vi "ConvertTdmsFileToNoDaqMxRaw.vi"() -> ()   [LabVIEW 2014]
panel:
  in  "转换总数":i64
  in  "偏移量":i64
  out "error":errorcluster
  in  "Convert":bool
  in  "Stop Button":bool
  in  "File With RawDaq":path
  in  "New File":path
  # "Very simple utility to read in a TDMS file and the write out to a new TDMS file.\nThis will strip out DAQmxRaw data which is problematic for reading with other tools."
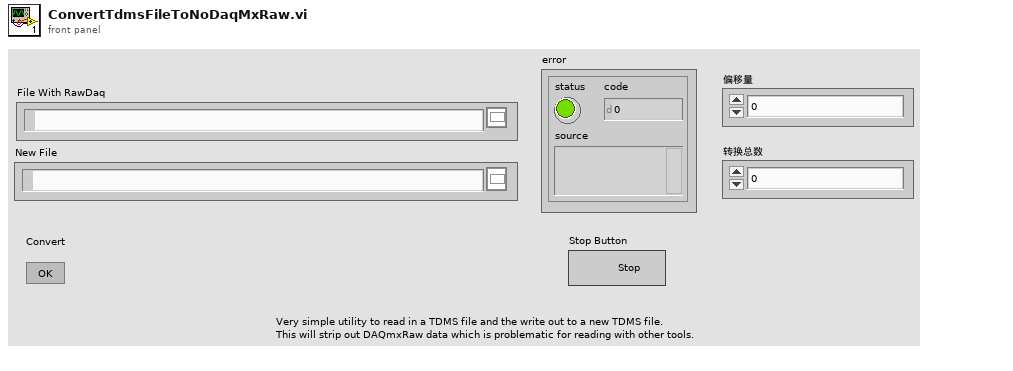
[diagram p1: front panel]
types:
  T1 = enum16{"open", "open or create", "create or replace", "create", "open (read-only)"}
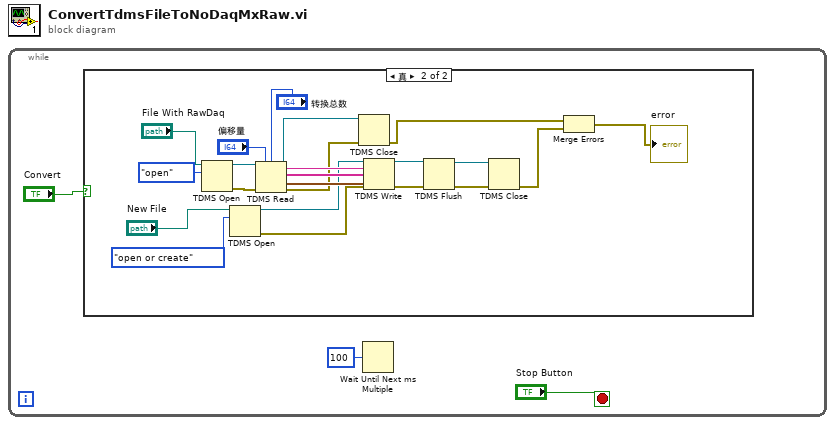
[diagram p0: block diagram]
diagram:
  n1 = while {
    stop <- "Stop Button" stop-if-true
    n2 = case shown="真" "Convert" {
      frame False {
      }
      frame True {
        n3 = TDMS Open(10:T1."open" ("operation (0:open)"), 11:"File With RawDaq") -> (0:w21:errorcluster, 3:w22:refnum<k34>)  [unwired: 5 in]
        n4 = TDMS Open(10:T1."open or create" ("operation (0:open)"), 11:"New File") -> (0:w9:errorcluster, 3:w18:refnum<k34>)  [unwired: 5 in]
        n5 = TDMS Read(0:w22, 1:"偏移量", 2:"转换总数", 11:w21) -> (4:w14:refnum<k34>, 6:w25:string, 8:w24:string[], 10:w23:waveform(dbl)[], 15:w15:errorcluster)  [unwired: 4 in, 1 out]
        n6 = TDMS Close(8:w15, 11:w14) -> (0:w8:errorcluster)  [unwired: 1 out]
        n7 = TDMS Write(0:w18, 5:w25, 7:w24, 9:w23, 11:w9) -> (4:w12:refnum<k34>, 15:w13:errorcluster)  [unwired: 1 in, 2 out]
        n8 = TDMS Flush(4:w13, 7:w12) -> (0:w11:errorcluster, 3:w10:refnum<k34>)
        n9 = TDMS Close(8:w11, 11:w10) -> (0:w7:errorcluster)  [unwired: 1 out]
        n10 = Merge Errors(w8, w7) -> (→"error":errorcluster)
      }
    }
    n11 = Wait Until Next ms Multiple(millisecond multiple=u32 100) -> ()  [unwired: 1 out]
  }
